vi "HRM-Stage3-Process_main.vi"(8 "error in (no error)":errorcluster, 11 "Init cluster":T1) -> (0 "error out":errorcluster)   [LabVIEW 2020]
uses:
  HRM-Stage3-init_cluster.ctl
  HRM-Stage3-User_events.ctl
  <vilib>/measure/matone.llb/Extract Single Tone Information 1 Chan.vi
  <vilib>/measure/NI_MAPro.lvlib
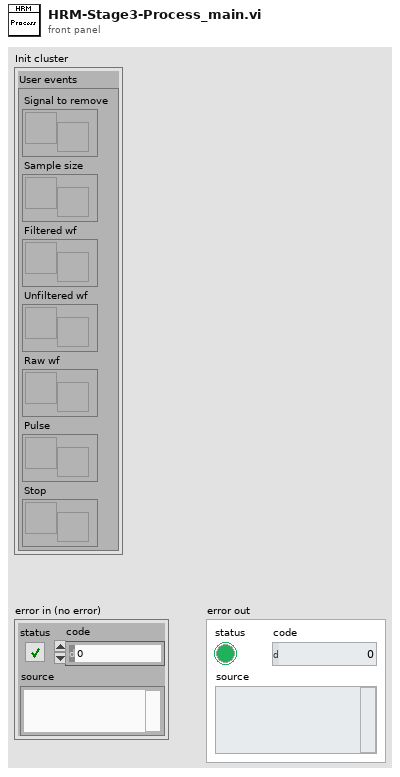
[diagram p1: front panel]
types:
  T1 = typedef "HRM-Stage3-init_cluster.ctl" = cluster{"User events":T2}
  T2 = typedef "HRM-Stage3-User_events.ctl" = cluster{"Signal to remove":refnum<user-event>, "Sample size":refnum<user-event>, "Filtered wf":refnum<user-event>, "Unfiltered wf":refnum<user-event>, "Raw wf":refnum<user-event>, "Pulse":refnum<user-event>, "Stop":refnum<user-event>}
  T3 = cluster{"Samples size (10)":i32, "Addition signal to remove":dbl, "Unfiltered wf":waveform(dbl), "User events":T2}
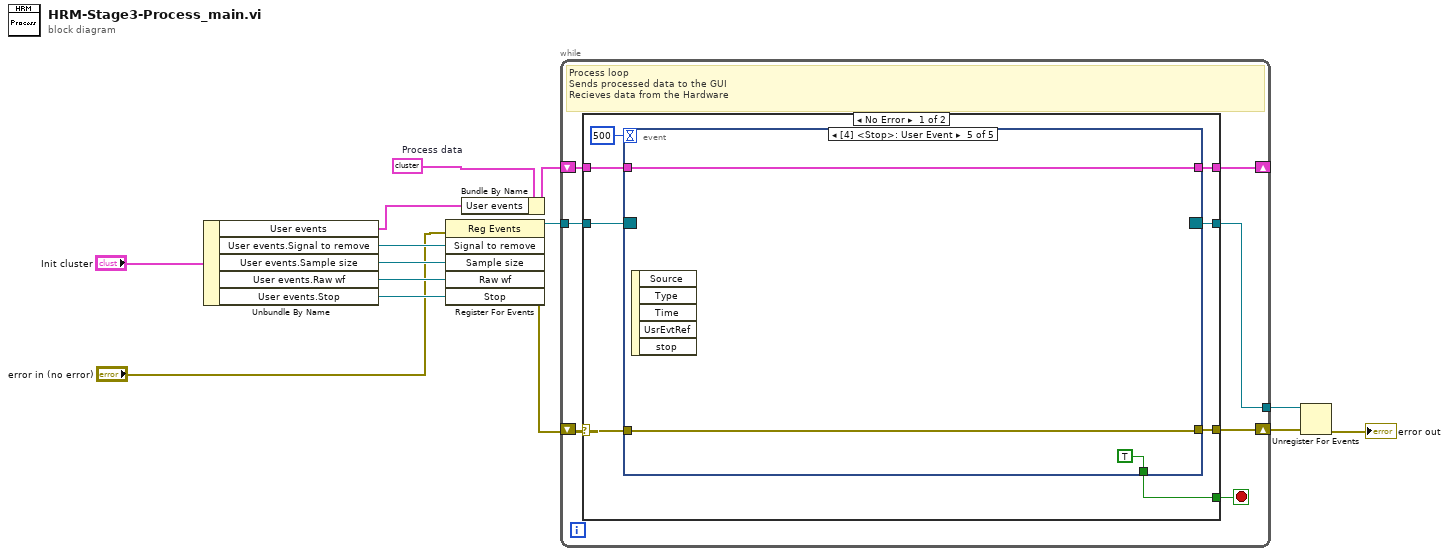
[diagram p0: block diagram]
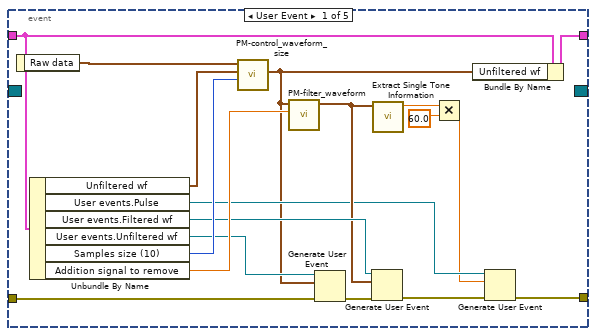
[diagram p2: hidden frame]
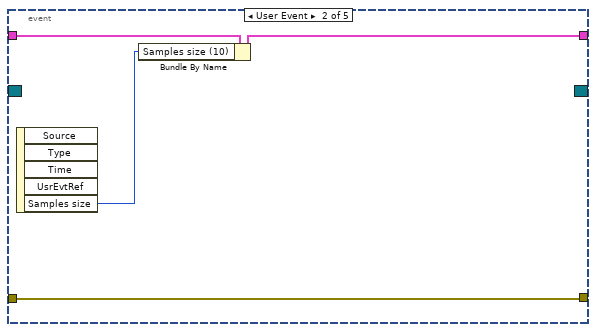
[diagram p3: hidden frame]
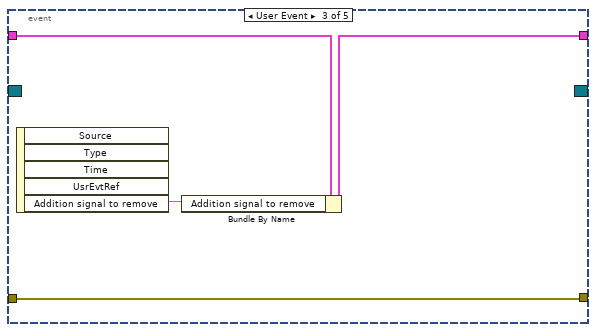
[diagram p4: hidden frame]
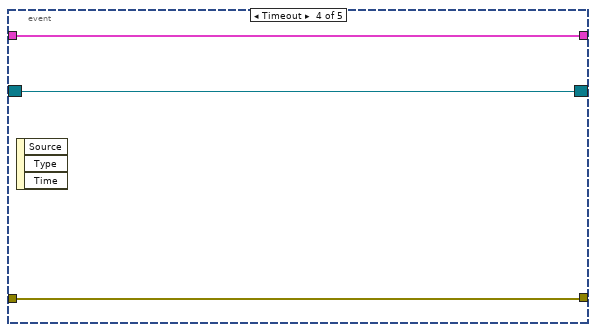
[diagram p5: hidden frame]
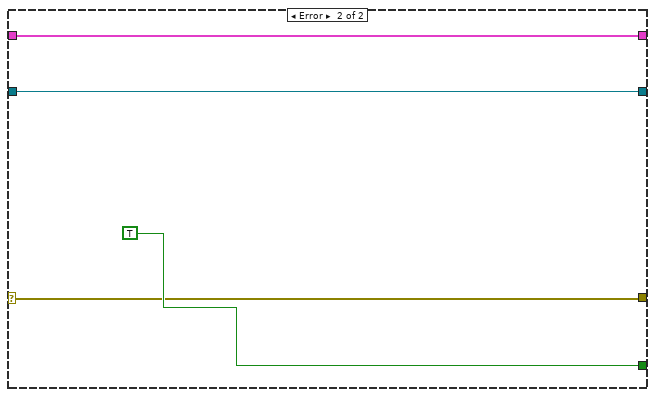
[diagram p6: hidden frame]
diagram:
  w3 = T3 {"Samples size (10)"=10, "Addition signal to remove"=0.0, "Unfiltered wf"={"t0"=timestamp(0 s since 1904-01-01), "dt"=1.0, "Y"=[]}, "User events"={"Signal to remove"=refnum, "Sample size"=refnum, "Filtered wf"=refnum, "Unfiltered wf"=refnum, "Raw wf"=refnum, "Pulse"=refnum, "Stop"=refnum}}  # Process data
  n1 = Unbundle By Name("Init cluster") -> ("User events"=w14:T2, "User events.Signal to remove"=w12:refnum<user-event>, "User events.Sample size"=w11:refnum<user-event>, "User events.Raw wf"=w10:refnum<user-event>, "User events.Stop"=w13:refnum<user-event>)
  n2 = register-events(error in="error in (no error)", w12, w11, w10, w13) -> (reference out=w2:refnum<event-registration>, error out=w1:errorcluster)  [unwired: 1 in]
  n3 = Bundle By Name(cluster=w3, "User events"=w14) -> (w4:T3)
  n4 = while {
    tunnel: w2 -> [w19]
    shift-right: [w17] -> _
    shift-left: w4 -> [w18]
    shift-right: [w16] -> w5
    shift-left: w1 -> [w20]
    tunnel: [w15] -> w6
    stop <- w21 stop-if-true
    # "Process loop\nSends processed data to the GUI\nRecieves data from the Hardware"
    n5 = case shown="No Error" w20 {
      selector: w20 -> [w26 w63]
      tunnel: [w22 TRUE ("Stop")] -> w21
      tunnel: w19 -> [w29 w62]
      tunnel: w18 -> [w28 w64]
      tunnel: [w27 w64] -> w17
      tunnel: [w25 w63] -> w16
      tunnel: [w23 w62] -> w15
      frame No Error {
        n6 = event shown="[4] <Stop>: User Event" {
          selector: w29 -> [_ _ _ w57 _]
          dyn-events: [_ _ _ w57 _] -> w23
          timeout: 500 -> [_ _ _ _ _]
          tunnel: w28 -> [w45 w51 w55 w58 w61]
          tunnel: [w34 w50 w54 w58 w61] -> w27
          tunnel: w26 -> [w31 w48 w52 w56 w59]
          tunnel: [w30 w48 w52 w56 w59] -> w25
          tunnel: [_ _ _ _ TRUE ("Stop")] -> w22
          event User Event {
            n7 = event-data() -> ("Raw data"=w46:waveform(dbl))  [unwired: 1 in]
            n8 = Unbundle By Name(w45) -> ("Unfiltered wf"=w32:waveform(dbl), "User events.Pulse"=w37:refnum<user-event>, "User events.Filtered wf"=w40:refnum<user-event>, "User events.Unfiltered wf"=w42:refnum<user-event>, "Samples size (10)"=w44:i32, "Addition signal to remove"=w43:dbl)
            n9 = call "PM-control_waveform_size.vi"("Samples s"=w44, "old waveform"=w32, "New waveform"=w46) -> ("waveform"=w33:waveform(dbl))  [unwired: 8 in]
            n10 = call "PM-filter_waveform.vi"("Addition signal to remove (0) [s]"=w43, "waveform in"=w33) -> ("waveform out"=w39:waveform(dbl))  [unwired: 8 in, 1 out]
            n11 = Generate User Event(user event=w42, event data cluster=w33, error in=w31) -> (error out=w41:errorcluster)  [unwired: 1 in, 1 out]
            n12 = Generate User Event(user event=w40, event data cluster=w39, error in=w41) -> (error out=w38:errorcluster)  [unwired: 1 in, 1 out]
            n13 = call-poly <vilib>:"Extract Single Tone Information.vi"("time signal in"=w39) -> ("detected frequency"=w36:dbl)  [unwired: 5 in, 5 out]
            n14 = Multiply(x=w36, y=60.0) -> (x*y=w35:dbl)
            n15 = Bundle By Name(cluster=w45, "Unfiltered wf"=w33) -> (w34:T3)
            n16 = Generate User Event(user event=w37, event data cluster=w35, error in=w38) -> (error out=w30:errorcluster)  [unwired: 1 in, 1 out]
          }
          event User Event {
            n17 = event-data() -> ("Samples size"=w49:i32)  [unwired: 1 in, 4 out]
            n18 = Bundle By Name(cluster=w51, "Samples size (10)"=w49) -> (w50:T3)
          }
          event User Event {
            n19 = event-data() -> ("Addition signal to remove"=w53:dbl)  [unwired: 1 in, 4 out]
            n20 = Bundle By Name(cluster=w55, "Addition signal to remove"=w53) -> (w54:T3)
          }
          event Timeout {
            n21 = event-data() -> ()  [unwired: 1 in, 3 out]
          }
          event User Event {
            n22 = event-data() -> ()  [unwired: 1 in, 5 out]
          }
        }
      }
      frame Error {
      }
    }
  }
  n23 = Unregister For Events(event registration refnum=w6, error in=w5) -> (error out=→"error out":errorcluster)
